vi "signalToGraphAndSpectrum(SubVI).vi"(0 "Vstupní signál":dbl[](array[numeric])) -> (1 "Signál do grafu":waveform(dbl)[](array[waveform]), 2 "Spektrum do grafu":cluster{"f0":dbl, "df":dbl, "magnitude":dbl[]}[](array[cluster]))   [LabVIEW 2025]
uses:
  <vilib>/measure/NI_MAPro.lvlib
  <vilib>/measure/maspectr.llb/FFT Spectrum (Mag-Phase) for 1 Chan.vi
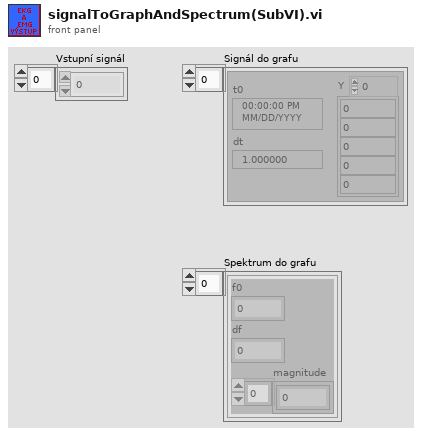
[diagram p1: front panel]
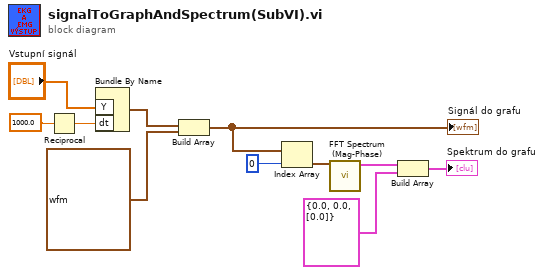
[diagram p0: block diagram]
diagram:
  n1 = Reciprocal(x=1000.0 ("dt")) -> (1/x=w3:dbl)
  n2 = Bundle By Name("Y"="Vstupní signál", "dt"=w3) -> (w4:waveform(dbl))  [unwired: 1 in]
  n3 = Build Array(w4, waveform(dbl) {"t0"=timestamp(0 s since 1904-01-01), "dt"=0.0, "Y"=[0.0]} ("element")) -> (w8:waveform(dbl)[])
  "Signál do grafu" <- w8
  n4 = Index Array(array=w8, index=0) -> (element=w7:waveform(dbl))
  n5 = call-poly <vilib>:"FFT Spectrum (Mag-Phase).vi"("time signal"=w7) -> ("magnitude"=w9:cluster{"f0":dbl, "df":dbl, "magnitude":dbl[]})  [unwired: 6 in, 4 out]
  n6 = Build Array(w9, cluster{"f0":dbl, "df":dbl, "magnitude":dbl[]} {"f0"=0.0, "df"=0.0, "magnitude"=[0.0]} ("element")) -> (→"Spektrum do grafu":cluster{"f0":dbl, "df":dbl, "magnitude":dbl[]}[])
